vi "Add Object to JSON Schema.vi"(8 "error in (no error)":errorcluster, 9 "Object":variant, 10 "Object Name":string, 11 "JSON Schema in":string) -> (0 "error out":errorcluster, 3 "JSON Schema out":string)   [LabVIEW 2019, in "JSON-Schema.lvlib"]
uses:
  JSON-Schema.lvlib
  <vilib>/JDP Science/JSONtext/JSONtext.lvlib
  <vilib>/Utility/Data Type/NI_Data Type.lvlib
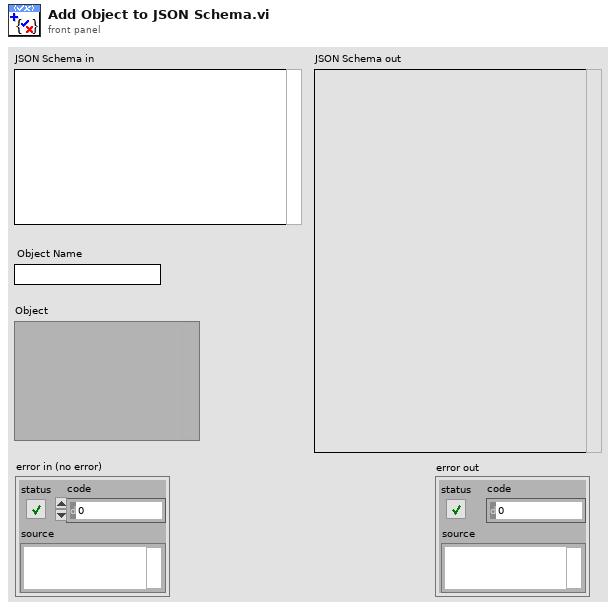
[diagram p1: front panel]
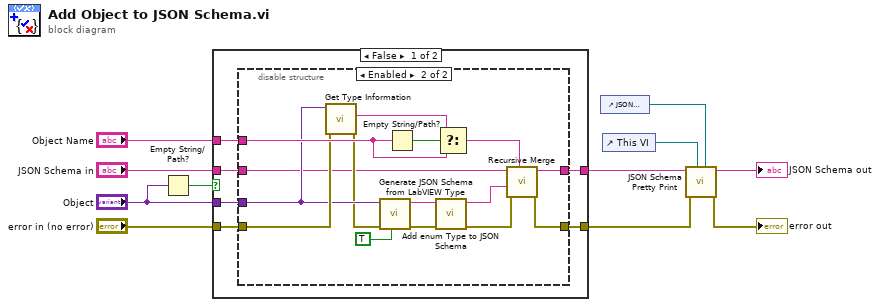
[diagram p0: block diagram]
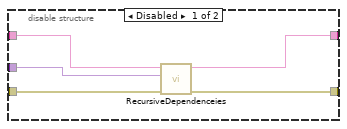
[diagram p2: hidden frame]
diagram:
  n1 = Empty String/Path?(string/path="Object") -> (empty?=w7:bool)
  n2 = case shown="False" w7 {
    tunnel: "error in (no error)" -> [w17 w39]
    tunnel: [w16 w38] -> w4
    tunnel: [w15 w39] -> w3
    tunnel: "Object Name" -> [w14 _]
    tunnel: "JSON Schema in" -> [w13 w38]
    tunnel: "Object" -> [w12 _]
    frame False {
      n3 = disable-structure shown="Enabled" {
        disable-tunnel: w12 -> [w22 w29]
        disable-tunnel: w17 -> [w21 w30]
        disable-tunnel: w13 -> [w20 w27]
        disable-tunnel: [w19 w35] -> w16
        disable-tunnel: [w18 w26] -> w15
        disable-tunnel: w14 -> [_ w32]
        frame Disabled {
          n4 = call "RecursiveDependenceies.vi"("error in (no error)"=w21, "Object"=w22, "JSON Schema in"=w20) -> ("error out"=w18:errorcluster, "JSON Schema out"=w19:string)  [unwired: 7 in]
        }
        frame Enabled {
          n5 = call <vilib>:"Get Type Information.vi"("error in (no error)"=w30, "variant"=w29) -> ("error out"=w28:errorcluster, "name"=w33:string)  [unwired: 5 in, 3 out]
          n6 = call <vilib>:"Generate JSON Schema from LabVIEW Type.vi"("Strict Clusters"=TRUE, "error in (no error)"=w28, "Variant"=w29) -> ("error out"=w37:errorcluster, "JSON Schema"=w36:string)  [unwired: 7 in]
          n7 = Empty String/Path?(string/path=w32) -> (empty?=w34:bool)
          n8 = call "Add enum Type to JSON Schema.vi"("error in (no error)"=w37, "JSON Schema in"=w36) -> ("error out"=w25:errorcluster, "JSON Schema out"=w24:string)  [unwired: 8 in]
          n9 = Select(t=w33, s=w34, f=w32) -> (s? t:f=w23:string)
          n10 = call "Recursive Merge.vi"("$Path or Item Name"=w23, "error in (no error)"=w25, "JSON Object to Merge"=w24, "JSON Schema in"=w27) -> ("error out"=w26:errorcluster, "JSON Schema out"=w35:string)  [unwired: 6 in]
        }
      }
    }
    frame True {
    }
  }
  n11 = control-ref of="JSON Schema out"() -> (w6:refnum<vi>)
  n12 = control-ref of="This VI"() -> (w5:refnum<vi>)
  n13 = call "JSON Schema Pretty Print.vi"("String Control"=w6, "reference"=w5, "error in (no error)"=w3, "<JSON> in"=w4) -> ("error out"=→"error out":errorcluster, "<JSON> out"=→"JSON Schema out":string)  [unwired: 6 in]
